vi "IVC_OC200_Main.vi"() -> ()   [LabVIEW 2019]
panel:
  out "Status":bool
  out "Last Meas. Time":timestamp format="%<%Y-%m-%d %H:%M:%S>T"
  out "chart":waveform(dbl)[](graph)=[{"t0"=timestamp(3785686355.130285 s since 1904-01-01), "dt"=1.0, "Y"=[-0.00251999]}, {"t0"=timestamp(3785686355.130285 s since 1904-01-01), "dt"=1.0, "Y"=[-0.00346989]}]
  out "CH2 (Torr)":dbl
  out "CH1 (Torr)":dbl
  in  "milliseconds to wait":u32=1000
  in  "stop":bool
  out "error out":errorcluster
  in  "VISA resource name":refnum<visa-resource-name>="COM41"
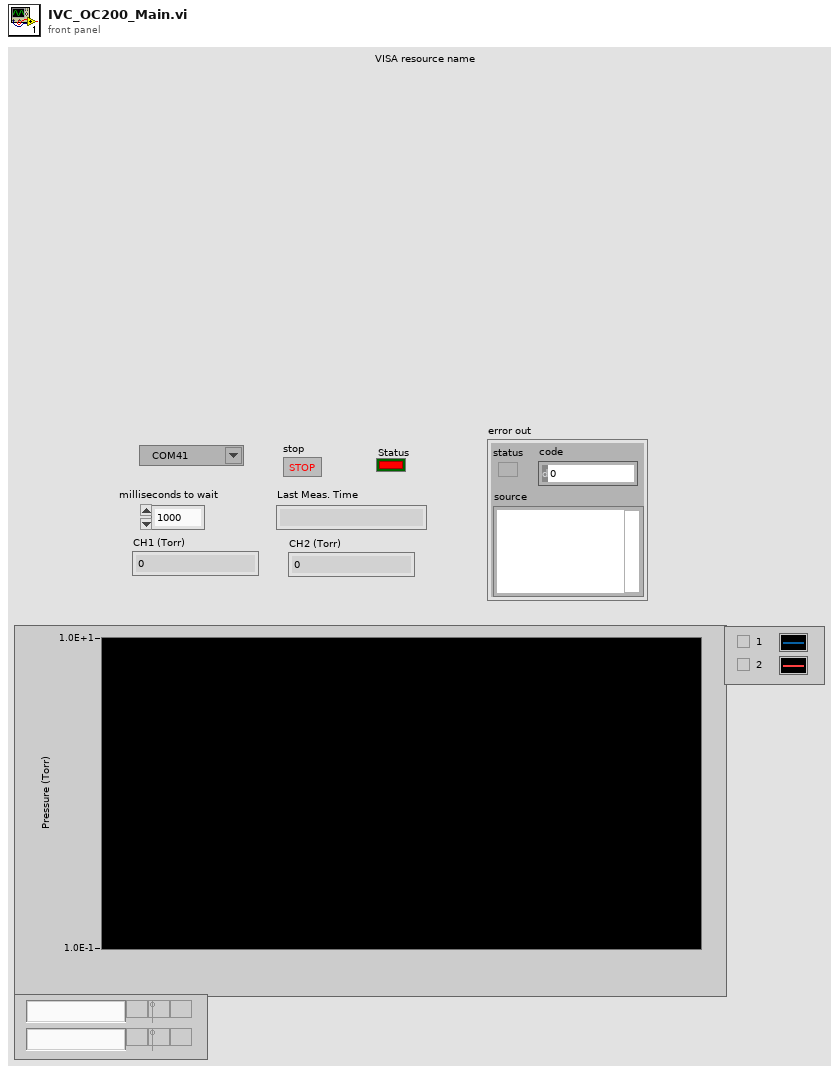
[diagram p1: front panel]
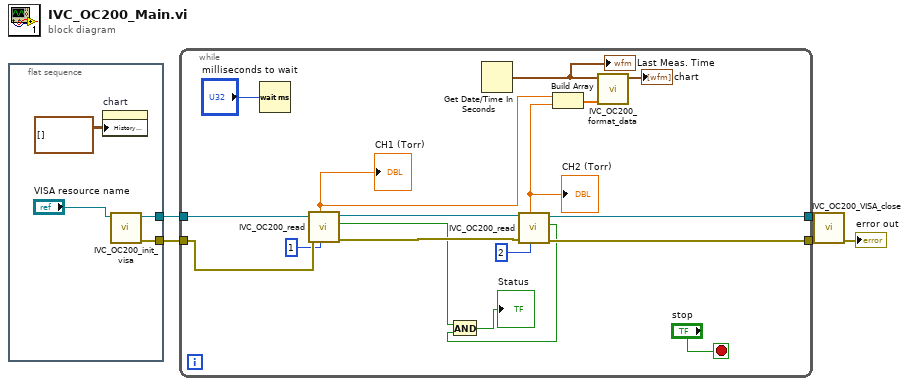
[diagram p0: block diagram]
diagram:
  n1 = flat-sequence {
    tunnel: [w8] -> w5
    tunnel: [w7] -> w4
    frame #0 {
      n2 = property on="chart" class="WFChart (strict)"("History Data"=waveform(dbl)[][] []) -> ()  [unwired: 2 in, 2 out]
      n3 = call "IVC_OC200_init_visa.vi"("VISA resource name"="VISA resource name") -> ("error out"=w7:errorcluster, "VISA resource name out"=w8:refnum<visa-resource-name>)  [unwired: 9 in]
    }
  }
  n4 = while {
    tunnel: w5 -> [w26]
    tunnel: w4 -> [w25]
    tunnel: [w22] -> w2
    tunnel: [w21] -> w1
    stop <- "stop" stop-if-true
    n5 = Wait (ms)(milliseconds to wait="milliseconds to wait") -> ()  [unwired: 1 out]
    n6 = call "IVC_OC200_read.vi"("Channel"=1, "error in (no error)"=w25, "VISA Refnum in"=w26) -> ("error out"=w20:errorcluster, "Status"=w12:bool, "VISA Refnum out"=w23:refnum<visa-resource-name>, "IVC (Torr)"=w19:dbl)  [unwired: 3 in, 2 out]
    "CH1 (Torr)" <- w19
    n7 = Get Date/Time In Seconds() -> (seconds since 1Jan1904=w15:timestamp)
    "Last Meas. Time" <- w15
    n8 = call "IVC_OC200_read.vi"("Channel"=2, "error in (no error)"=w20, "VISA Refnum in"=w23) -> ("error out"=w22:errorcluster, "Status"=w11:bool, "VISA Refnum out"=w21:refnum<visa-resource-name>, "IVC (Torr)"=w18:dbl)  [unwired: 3 in, 2 out]
    "CH2 (Torr)" <- w18
    n9 = And(x=w12, y=w11) -> (x .and. y?=→"Status":bool)
    n10 = Build Array(w19, w18) -> (w17:dbl[])
    n11 = call "IVC_OC200_format_data.vi"("element"=w17, "time"=w15) -> ("waveform_array_A"=→"chart":waveform(dbl)[])  [unwired: 9 in]
  }
  n12 = call "IVC_OC200_VISA_close.vi"("error in (no error)"=w2, "VISA resource name"=w1) -> ("error out"=→"error out":errorcluster)  [unwired: 9 in]
